vi "Waveform Width.vi"(10 "Threshold":dbl, 11 "Waveform":i16[](array[numeric])) -> (3 "Width (in samples)":i32)   [LabVIEW 2011]
uses:
  <vilib>/Analysis/NI_AALPro.lvlib
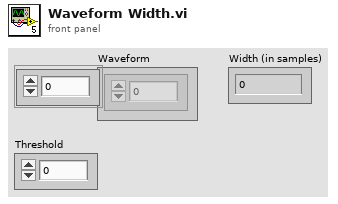
[diagram p1: front panel]
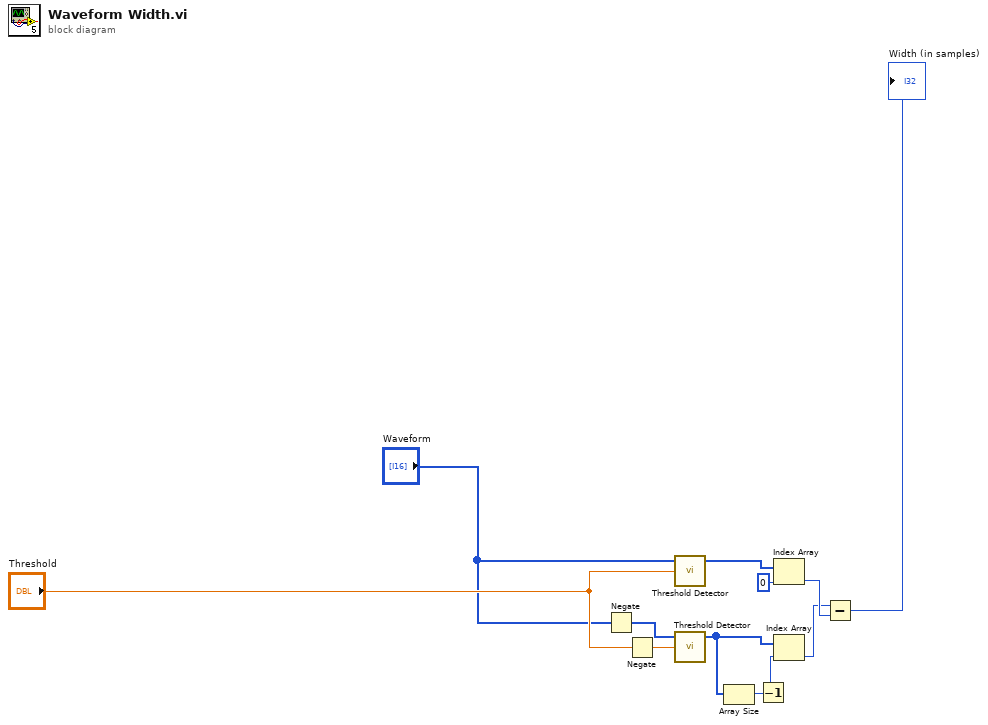
[diagram p0: block diagram]
diagram:
  n1 = Negate(x="Waveform") -> (-x=w4:i16[])
  n2 = Negate(x="Threshold") -> (-x=w6:dbl)
  n3 = call <vilib>:"Threshold Detector.vi"("threshold"="Threshold", "X"="Waveform") -> ("Indices"=w8:i32[])  [unwired: 1 in, 2 out]
  n4 = call <vilib>:"Threshold Detector.vi"("threshold"=w6, "X"=w4) -> ("Indices"=w3:i32[])  [unwired: 1 in, 2 out]
  n5 = Array Size(array=w3) -> (size(s)=w1:i32)
  n6 = Decrement(x=w1) -> (x-1=w2:i32)
  n7 = Index Array(array=w8, index=0) -> (element=w11:i32)
  n8 = Index Array(array=w3, index=w2) -> (element=w10:i32)
  n9 = Subtract(x=w10, y=w11) -> (x-y=→"Width (in samples)":i32)
